vi "Shooter_Operator_Assist.vi"(0 "Turret Aimed":bool, 5 "Ball In Position":bool, 7 "Shooter Motor Speed Good":bool, 9 "Shoot Command":bool, 11 "Start":bool) -> (4 "BottomFeeder":bool=TRUE, 6 "ShooterMotor":bool=TRUE, 8 "TurretMotor":bool=TRUE, 10 "TopFeeder":bool=TRUE)   [LabVIEW 2016]
panel:
  in  "ShooterState":enum16{"Idle", "Recover", "Shoot", "QueueFuel"}(ring)
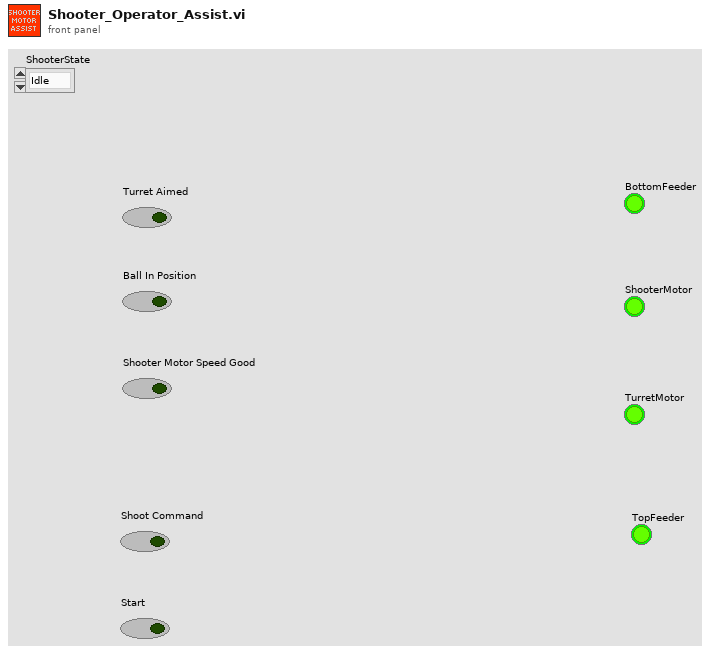
[diagram p1: front panel]
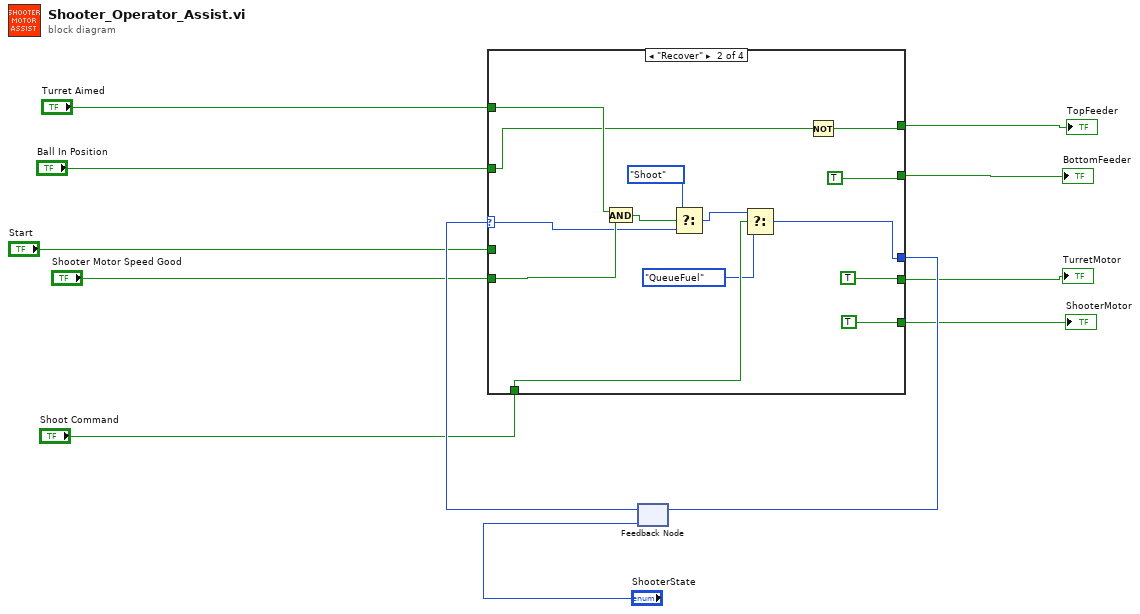
[diagram p0: block diagram]
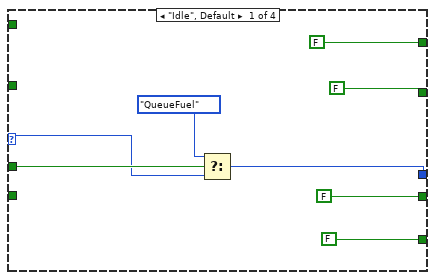
[diagram p2: hidden frame]
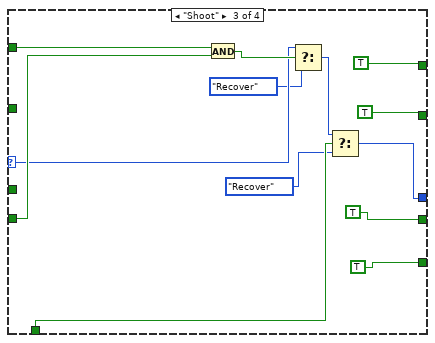
[diagram p3: hidden frame]
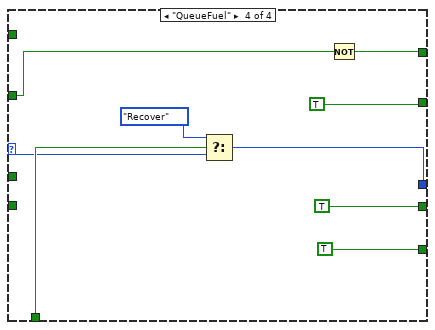
[diagram p4: hidden frame]
diagram:
  n1 = feedback #1("ShooterState") -> (w11:enum16{"Idle", "Recover", "Shoot", "QueueFuel"})
  n2 = case shown="\"Recover\"" w11 {
    selector: w11 -> [w19 w31 w44 w55]
    tunnel: [w18 w28 w39 w53] -> w9
    tunnel: "Start" -> [w20 _ _ _]
    tunnel: "Shoot Command" -> [_ w27 w42 w56]
    tunnel: "Shooter Motor Speed Good" -> [_ w34 w45 _]
    tunnel: "Turret Aimed" -> [_ w33 w47 _]
    tunnel: "Ball In Position" -> [_ w25 _ w48]
    tunnel: [FALSE w24 TRUE w49] -> w4
    tunnel: [FALSE TRUE TRUE TRUE] -> w3
    tunnel: [FALSE TRUE TRUE TRUE] -> w2
    tunnel: [FALSE TRUE TRUE TRUE] -> w1
    frame "Idle", Default {
      n3 = Select(t=enum16{"Idle", "Recover", "Shoot", "QueueFuel"}."QueueFuel", s=w20, f=w19) -> (s? t:f=w18:enum16{"Idle", "Recover", "Shoot", "QueueFuel"})
    }
    frame "Recover" {
      n4 = And(x=w33, y=w34) -> (x .and. y?=w32:bool)
      n5 = Select(t=enum16{"Idle", "Recover", "Shoot", "QueueFuel"}."Shoot", s=w32, f=w31) -> (s? t:f=w29:enum16{"Idle", "Recover", "Shoot", "QueueFuel"})
      n6 = Select(t=w29, s=w27, f=enum16{"Idle", "Recover", "Shoot", "QueueFuel"}."QueueFuel") -> (s? t:f=w28:enum16{"Idle", "Recover", "Shoot", "QueueFuel"})
      n7 = Not(x=w25) -> (.not. x?=w24:bool)
    }
    frame "Shoot" {
      n8 = And(x=w47, y=w45) -> (x .and. y?=w46:bool)
      n9 = Select(t=w44, s=w46, f=enum16{"Idle", "Recover", "Shoot", "QueueFuel"}."Recover") -> (s? t:f=w41:enum16{"Idle", "Recover", "Shoot", "QueueFuel"})
      n10 = Select(t=w41, s=w42, f=enum16{"Idle", "Recover", "Shoot", "QueueFuel"}."Recover") -> (s? t:f=w39:enum16{"Idle", "Recover", "Shoot", "QueueFuel"})
    }
    frame "QueueFuel" {
      n11 = Select(t=enum16{"Idle", "Recover", "Shoot", "QueueFuel"}."Recover", s=w56, f=w55) -> (s? t:f=w53:enum16{"Idle", "Recover", "Shoot", "QueueFuel"})
      n12 = Not(x=w48) -> (.not. x?=w49:bool)
    }
  }
  "TopFeeder" <- w4
  "BottomFeeder" <- w3
  "TurretMotor" <- w2
  "ShooterMotor" <- w1
  n13 = feedback-in #1(w9) -> ()
